vi "path_Forward.vi"() -> ()   [LabVIEW 2019]
uses:
  WSCbot_V3_Toolkit.lvlibp
panel:
  out "Hight":i32
  out "finish?":bool
  in  "Stop Button":bool
  in  "get the screw\n(XYZ)":cluster{"X":dbl, "Y":dbl, "Z":dbl}[](array[cluster])=[{"X"=-132.0, "Y"=15.0, "Z"=180.0}, {"X"=0.0, "Y"=0.0, "Z"=0.0}, {"X"=0.0, "Y"=0.0, "Z"=0.0}, {"X"=0.0, "Y"=0.0, "Z"=0.0}]
  in  "go to start\n(XYZ)":cluster{"X":dbl, "Y":dbl, "Z":dbl}[](array[cluster])=[{"X"=0.0, "Y"=-295.0, "Z"=0.0}, {"X"=0.0, "Y"=0.0, "Z"=0.0}, {"X"=0.0, "Y"=0.0, "Z"=0.0}, {"X"=0.0, "Y"=0.0, "Z"=0.0}]
  in  "go to showstage\n(XYZ)":cluster{"X":dbl, "Y":dbl, "Z":dbl}[](array[cluster])=[{"X"=0.0, "Y"=60.0, "Z"=0.0}, {"X"=0.0, "Y"=0.0, "Z"=0.0}, {"X"=0.0, "Y"=0.0, "Z"=0.0}, {"X"=0.0, "Y"=0.0, "Z"=0.0}]
  in  "cross hill\n(XYZ)":cluster{"X":dbl, "Y":dbl, "Z":dbl}[](array[cluster])=[{"X"=85.0, "Y"=0.0, "Z"=0.0}, {"X"=2.5, "Y"=140.0, "Z"=0.0}, {"X"=85.0, "Y"=0.0, "Z"=0.0}, {"X"=0.0, "Y"=0.0, "Z"=0.0}]
  in  "Get the nut\n(XYZ)":cluster{"X":dbl, "Y":dbl, "Z":dbl}[](array[cluster])=[{"X"=0.0, "Y"=-195.0, "Z"=180.0}, {"X"=0.0, "Y"=-100.0, "Z"=0.0}, {"X"=0.0, "Y"=0.0, "Z"=0.0}, {"X"=0.0, "Y"=0.0, "Z"=0.0}]
  in  "Back to start\n(XYZ)":cluster{"X":dbl, "Y":dbl, "Z":dbl}[](array[cluster])=[{"X"=0.0, "Y"=-300.0, "Z"=0.0}, {"X"=0.0, "Y"=0.0, "Z"=0.0}, {"X"=0.0, "Y"=0.0, "Z"=0.0}, {"X"=0.0, "Y"=0.0, "Z"=0.0}]
  in  "re_cross hill\n(XYZ)":cluster{"X":dbl, "Y":dbl, "Z":dbl}[](array[cluster])=[{"X"=70.0, "Y"=0.0, "Z"=0.0}, {"X"=0.0, "Y"=145.0, "Z"=0.0}, {"X"=75.0, "Y"=0.0, "Z"=0.0}, {"X"=0.0, "Y"=60.0, "Z"=0.0}]
  in  "Get nut\n(XYZ)":cluster{"X":dbl, "Y":dbl, "Z":dbl}[](array[cluster])=[{"X"=0.0, "Y"=125.0, "Z"=0.0}, {"X"=0.0, "Y"=-125.0, "Z"=0.0}, {"X"=0.0, "Y"=0.0, "Z"=0.0}]
  in  "Cross hill\n(XYZ)":cluster{"X":dbl, "Y":dbl, "Z":dbl}[](array[cluster])=[{"X"=-85.0, "Y"=0.0, "Z"=0.0}, {"X"=-5.0, "Y"=-140.0, "Z"=0.0}, {"X"=-75.0, "Y"=0.0, "Z"=0.0}]
  in  "go to hill\n(XYZ)":cluster{"X":dbl, "Y":dbl, "Z":dbl}[](array[cluster])=[{"X"=150.0, "Y"=0.0, "Z"=0.0}, {"X"=0.0, "Y"=-55.0, "Z"=0.0}, {"X"=0.0, "Y"=0.0, "Z"=0.0}]
  in  "Get screw\n(XYZ)":cluster{"X":dbl, "Y":dbl, "Z":dbl}[](array[cluster])=[{"X"=-10.0, "Y"=35.0, "Z"=-45.0}, {"X"=0.0, "Y"=0.0, "Z"=45.0}, {"X"=0.0, "Y"=270.0, "Z"=0.0}, {"X"=-150.0, "Y"=0.0, "Z"=0.0}]
  in  "Error In":errorcluster
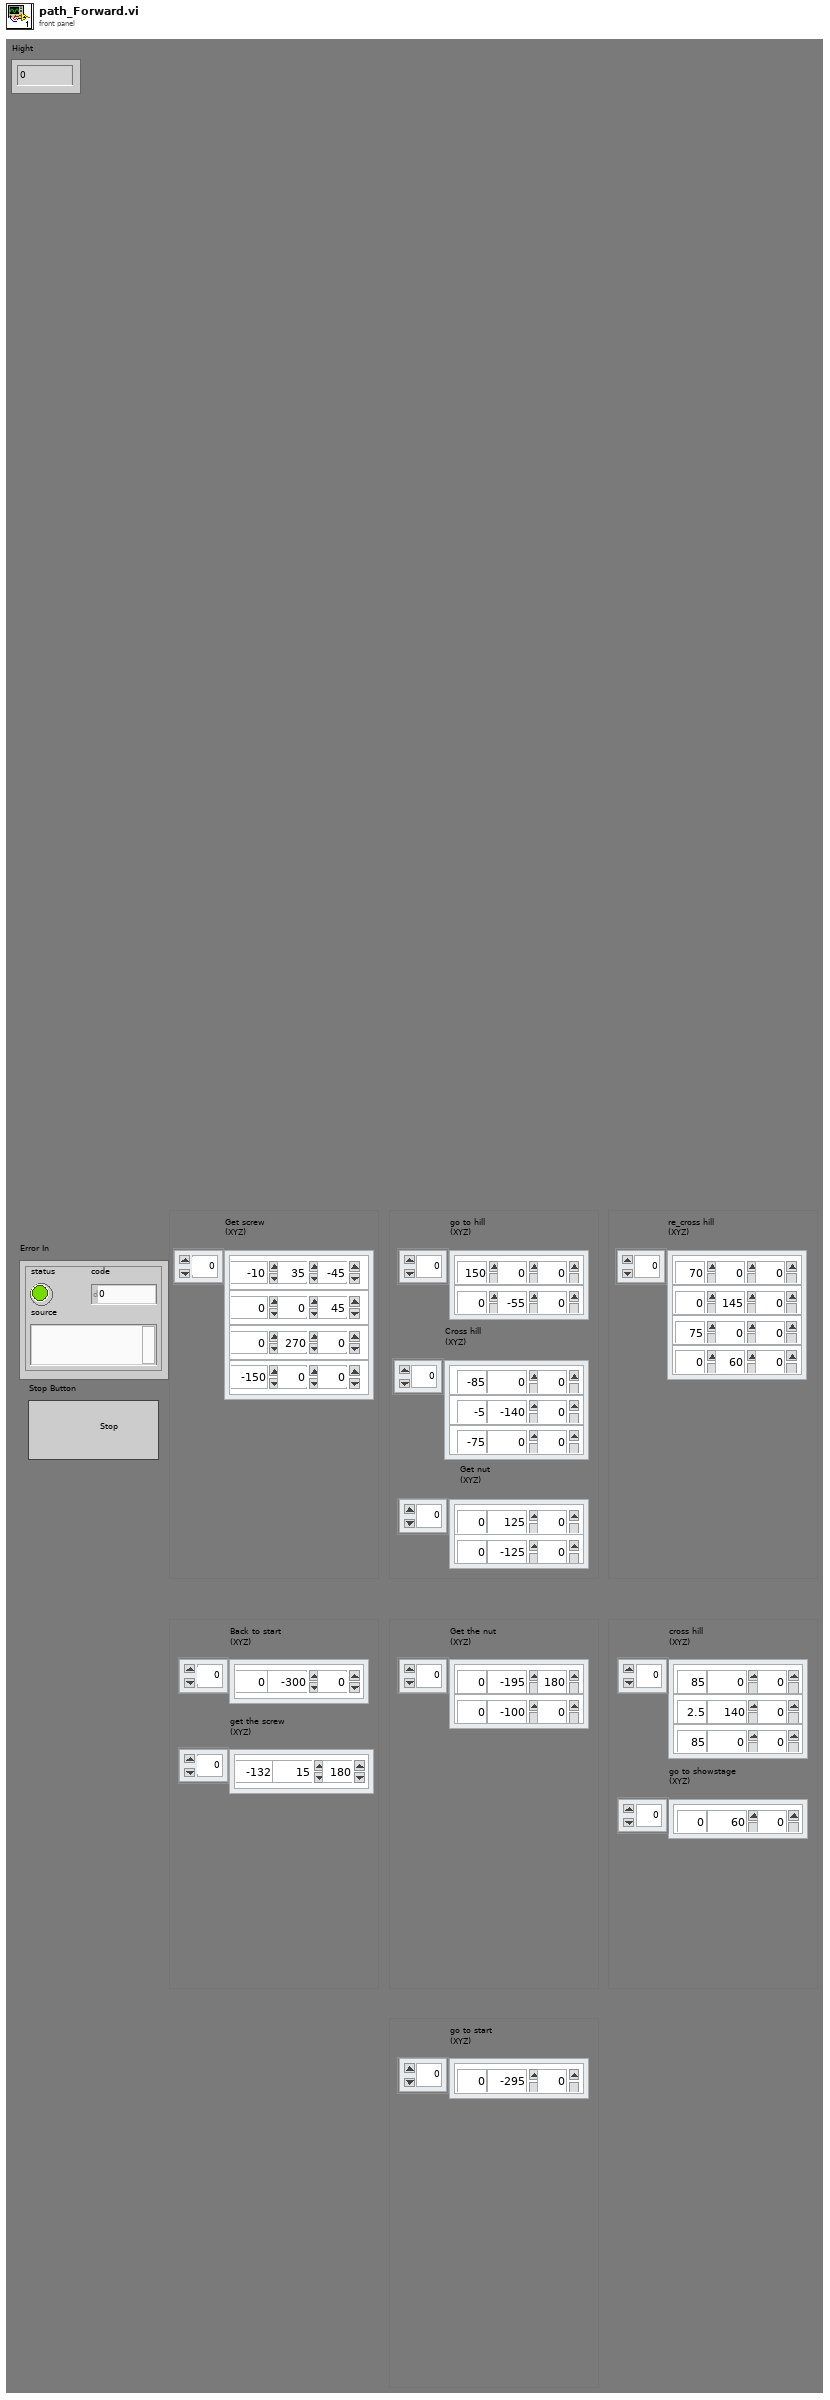
[diagram p1: front panel]
types:
  T1 = enum16{"Right_up", "Right_down", "Left_down", "Left_up", "left", "right", "up", "down"}
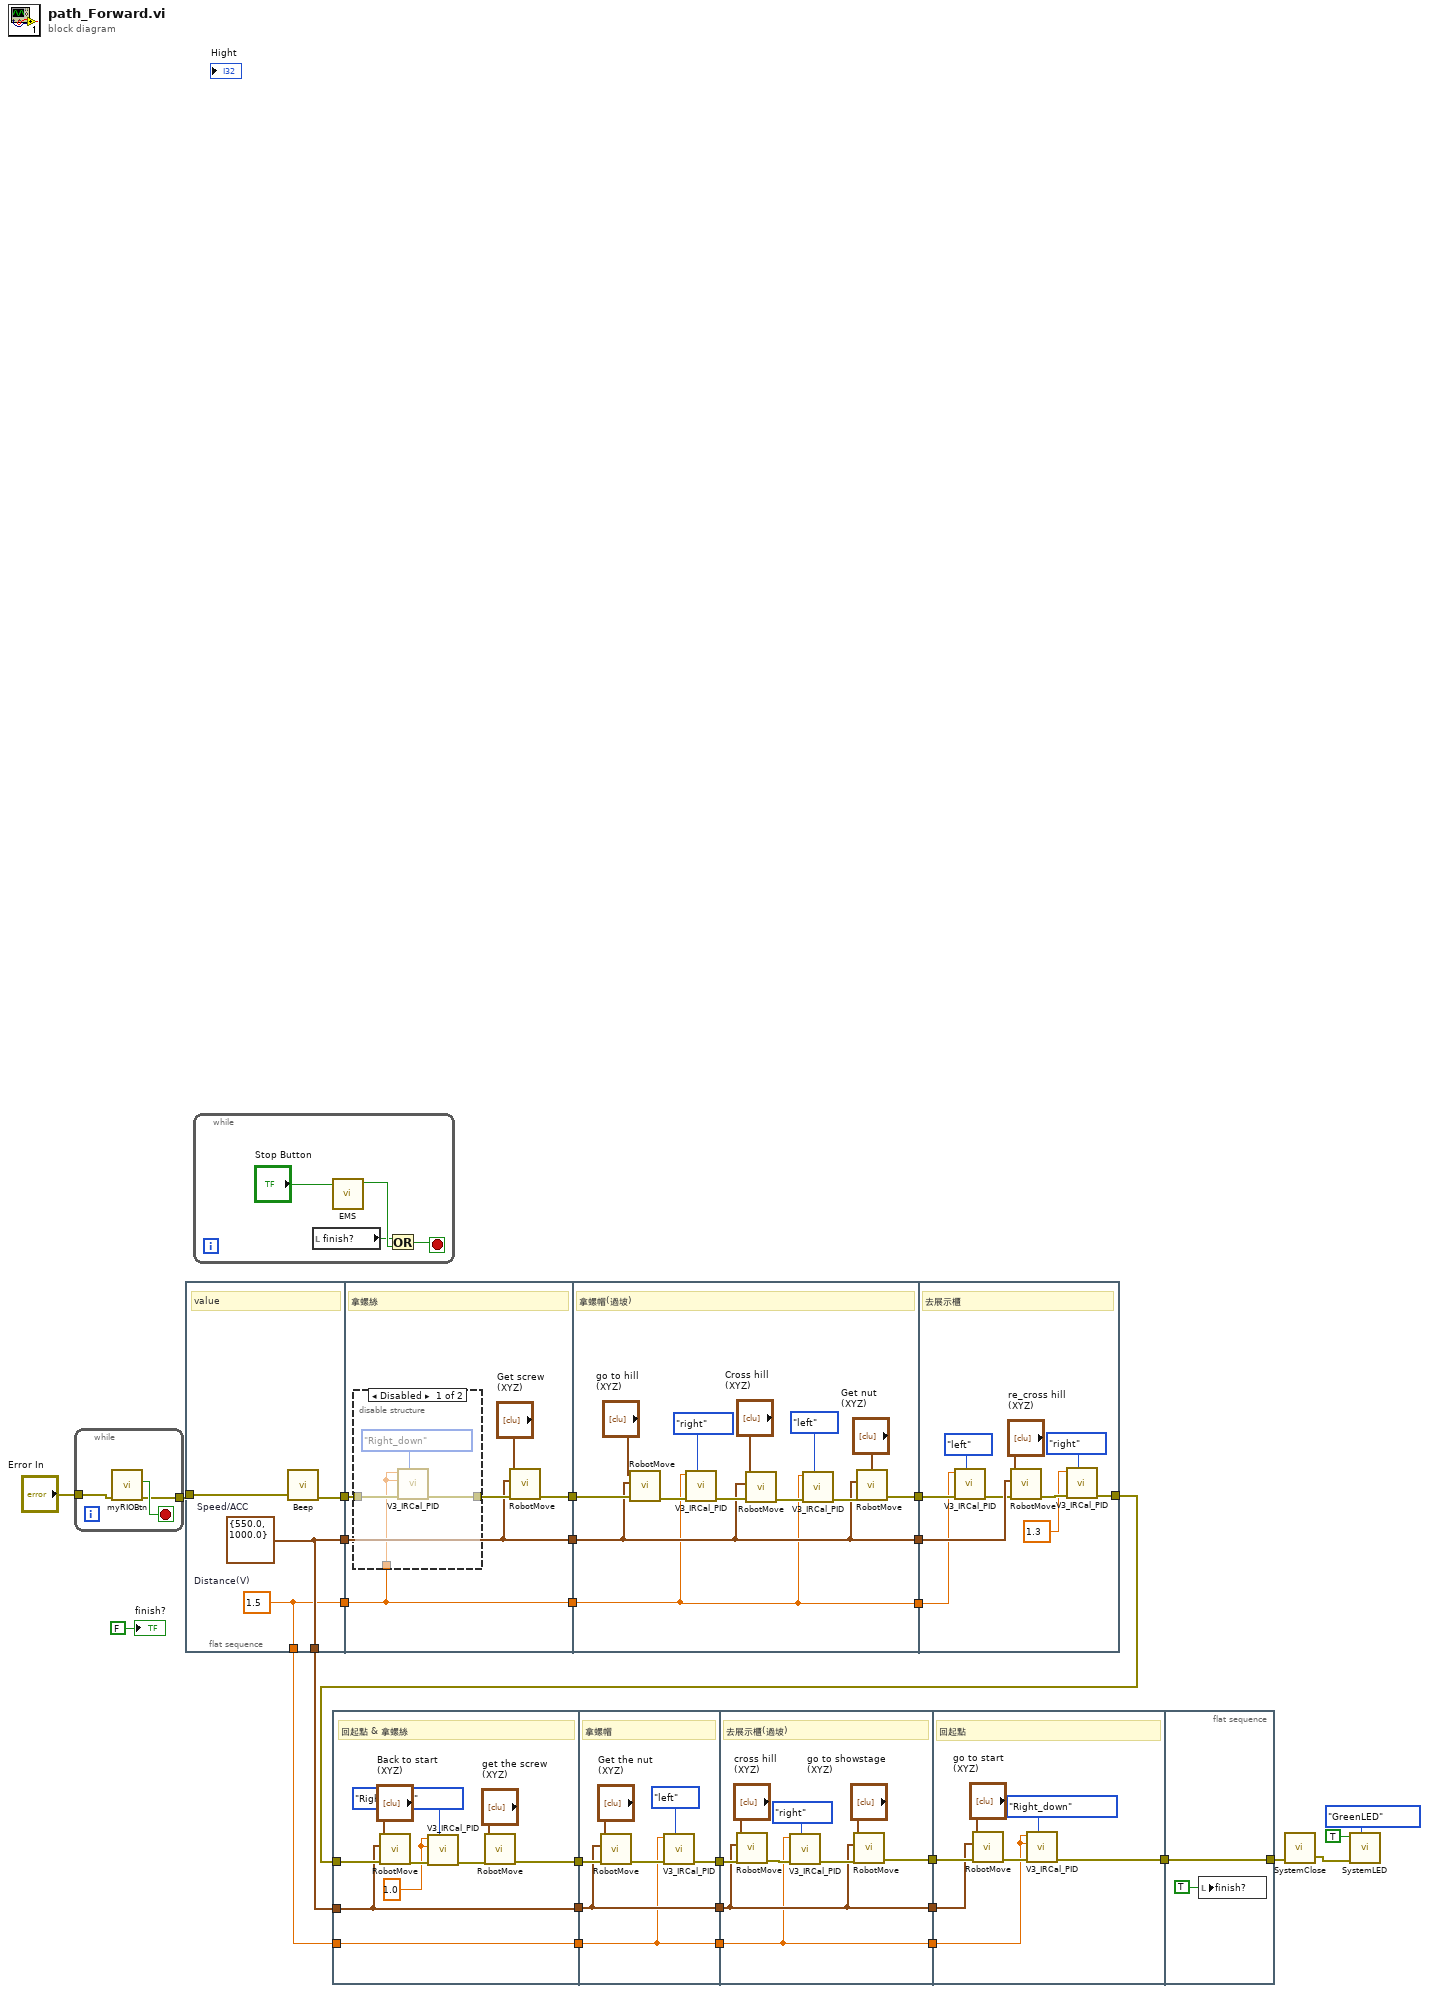
[diagram p0: block diagram]
diagram:
  n1 = while {
    tunnel: "Error In" -> [w31]
    tunnel: [w30] -> w2
    stop <- w32 stop-if-true
    n2 = call "myRIOBtn.vi"("error in"=w31) -> ("error out"=w30:errorcluster, "myRIOButton"=w32:bool)  [unwired: 9 in]
  }
  n3 = flat-sequence {
    tunnel: [w36] -> w29
    tunnel: [w34] -> w28
    tunnel: [w35] -> w25
    tunnel: [w36] -> w19
    tunnel: [w35] -> w18
    tunnel: w2 -> [w33]
    tunnel: w29 -> [w38]
    tunnel: w28 -> [w42]
    tunnel: [w39] -> w27
    tunnel: [w38] -> w26
    tunnel: w25 -> [w37]
    tunnel: [w37] -> w24
    tunnel: w27 -> [w59]
    tunnel: w26 -> [w48]
    tunnel: w24 -> [w47]
    tunnel: [w49] -> w23
    tunnel: [w48] -> w22
    tunnel: [w47] -> w21
    tunnel: w23 -> [w67]
    tunnel: w22 -> [w69]
    tunnel: w21 -> [w62]
    tunnel: [w61] -> w20
    frame #0 {
      w35 = 1.5  # Distance(V)
      w36 = cluster{dbl, dbl} {550.0, 1000.0}  # Speed/ACC
      # "value"
      n4 = call "Beep.vi"("Error In"=w33) -> ("Error Out"=w34:errorcluster)  [unwired: 10 in]
    }
    frame #1 {
      # "拿螺絲"
      n5 = disable-structure shown="Disabled" {
        disable-tunnel: w42 -> [w45 _]
        disable-tunnel: [w44 _] -> w40
        disable-tunnel: w37 -> [w43 _]
        frame Disabled {
          n6 = call "V3_IRCal_PID.vi"("Direction"=T1."Right_down", "Error In"=w45, "Y_distance(V)"=w43, "X_distance(V)"=w43) -> ("Error Out"=w44:errorcluster)  [unwired: 6 in, 1 out]
        }
        frame Enabled {
        }
      }
      n7 = call "RobotMove.vi"("error in (no error)"=w40, "Speed/ACC"=w38, "XYZ"="Get screw\n(XYZ)") -> ("error out"=w39:errorcluster)  [unwired: 8 in]
    }
    frame #2 {
      # "拿螺帽(過坡)"
      n8 = call "RobotMove.vi"("error in (no error)"=w59, "Speed/ACC"=w48, "XYZ"="go to hill\n(XYZ)") -> ("error out"=w57:errorcluster)  [unwired: 8 in]
      n9 = call "V3_IRCal_PID.vi"("Direction"=T1."right", "Error In"=w57, "X_distance(V)"=w47) -> ("Error Out"=w55:errorcluster)  [unwired: 7 in, 1 out]
      n10 = call "RobotMove.vi"("error in (no error)"=w55, "Speed/ACC"=w48, "XYZ"="Cross hill\n(XYZ)") -> ("error out"=w53:errorcluster)  [unwired: 8 in]
      n11 = call "V3_IRCal_PID.vi"("Direction"=T1."left", "Error In"=w53, "X_distance(V)"=w47) -> ("Error Out"=w51:errorcluster)  [unwired: 7 in, 1 out]
      n12 = call "RobotMove.vi"("error in (no error)"=w51, "Speed/ACC"=w48, "XYZ"="Get nut\n(XYZ)") -> ("error out"=w49:errorcluster)  [unwired: 8 in]
    }
    frame #3 {
      # "去展示櫃"
      n13 = call "V3_IRCal_PID.vi"("Direction"=T1."left", "Error In"=w67, "X_distance(V)"=w62) -> ("Error Out"=w68:errorcluster)  [unwired: 7 in, 1 out]
      n14 = call "RobotMove.vi"("error in (no error)"=w68, "Speed/ACC"=w69, "XYZ"="re_cross hill\n(XYZ)") -> ("error out"=w64:errorcluster)  [unwired: 8 in]
      n15 = call "V3_IRCal_PID.vi"("Direction"=T1."right", "Error In"=w64, "X_distance(V)"=1.3) -> ("Error Out"=w61:errorcluster)  [unwired: 7 in, 1 out]
    }
  }
  n16 = while {
    stop <- w72 stop-if-true
    n17 = local read "finish?"() -> (w70:bool)
    n18 = call "EMS.vi"("ProgramStop"="Stop Button") -> ("EMS"=w71:bool)  [unwired: 9 in, 1 out]
    n19 = Or(x=w70, y=w71) -> (x .or. y?=w72:bool)
  }
  n20 = flat-sequence {
    tunnel: w20 -> [w82]
    tunnel: w19 -> [w80]
    tunnel: w18 -> [w75]
    tunnel: [w78] -> w17
    tunnel: [w80] -> w16
    tunnel: [w75] -> w15
    tunnel: w17 -> [w89]
    tunnel: w16 -> [w85]
    tunnel: w15 -> [w84]
    tunnel: [w86] -> w14
    tunnel: [w85] -> w13
    tunnel: [w84] -> w12
    tunnel: w14 -> [w98]
    tunnel: w13 -> [w92]
    tunnel: w12 -> [w91]
    tunnel: [w93] -> w11
    tunnel: [w92] -> w10
    tunnel: [w91] -> w9
    tunnel: w11 -> [w105]
    tunnel: w10 -> [w104]
    tunnel: w9 -> [w102]
    tunnel: [w100] -> w4
    tunnel: [w108] -> w8
    tunnel: w4 -> [w108]
    frame #0 {
      w74 = 1.0 ("X_distance(V)")
      # "回起點 & 拿螺絲"
      n21 = call "RobotMove.vi"("error in (no error)"=w82, "Speed/ACC"=w80, "XYZ"="Back to start\n(XYZ)") -> ("error out"=w76:errorcluster)  [unwired: 8 in]
      n22 = call "V3_IRCal_PID.vi"("Direction"=T1."Right_down", "Error In"=w76, "Y_distance(V)"=w74, "X_distance(V)"=w74) -> ("Error Out"=w77:errorcluster)  [unwired: 6 in, 1 out]
      n23 = call "RobotMove.vi"("error in (no error)"=w77, "XYZ"="get the screw\n(XYZ)") -> ("error out"=w78:errorcluster)  [unwired: 9 in]
    }
    frame #1 {
      # "拿螺帽"
      n24 = call "RobotMove.vi"("error in (no error)"=w89, "Speed/ACC"=w85, "XYZ"="Get the nut\n(XYZ)") -> ("error out"=w88:errorcluster)  [unwired: 8 in]
      n25 = call "V3_IRCal_PID.vi"("Direction"=T1."left", "Error In"=w88, "X_distance(V)"=w84) -> ("Error Out"=w86:errorcluster)  [unwired: 7 in, 1 out]
    }
    frame #2 {
      # "去展示櫃(過坡)"
      n26 = call "RobotMove.vi"("error in (no error)"=w98, "Speed/ACC"=w92, "XYZ"="cross hill\n(XYZ)") -> ("error out"=w96:errorcluster)  [unwired: 8 in]
      n27 = call "V3_IRCal_PID.vi"("Direction"=T1."right", "Error In"=w96, "X_distance(V)"=w91) -> ("Error Out"=w94:errorcluster)  [unwired: 7 in, 1 out]
      n28 = call "RobotMove.vi"("error in (no error)"=w94, "Speed/ACC"=w92, "XYZ"="go to showstage\n(XYZ)") -> ("error out"=w93:errorcluster)  [unwired: 8 in]
    }
    frame #3 {
      # "回起點"
      n29 = call "RobotMove.vi"("error in (no error)"=w105, "Speed/ACC"=w104, "XYZ"="go to start\n(XYZ)") -> ("error out"=w103:errorcluster)  [unwired: 8 in]
      n30 = call "V3_IRCal_PID.vi"("Direction"=T1."Right_down", "Error In"=w103, "Y_distance(V)"=w102, "X_distance(V)"=w102) -> ("Error Out"=w100:errorcluster)  [unwired: 6 in, 1 out]
    }
    frame #4 {
      n31 = local write "finish?"(TRUE ("finish?")) -> ()
    }
  }
  n32 = call "SystemClose.vi"("error in"=w8) -> ("error out"=w7:errorcluster)  [unwired: 2 in]
  n33 = call "SystemLED.vi"("SelectColor"=enum16{"RedLED", "GreenLED", "YellowLED"}."GreenLED", "error in"=w7, "Set"=TRUE) -> ()  [unwired: 8 in, 1 out]
  "finish?" <- FALSE ("finish?")
